vi "Handle Error.vi"(8 "error in (no error)":errorcluster, 11 "BNT_DAQmx-MCSV-AIAvg in":refnum<class "BNT_DAQmx-MCSV-AIAvg.lvclass">) -> (0 "error out":errorcluster, 2 "stop actor?":bool=TRUE, 3 "BNT_DAQmx-MCSV-AIAvg out":refnum<class "BNT_DAQmx-MCSV-AIAvg.lvclass">)   [LabVIEW 2019, in "BNT_DAQmx.lvlib" / "BNT_DAQmx-MCSV-AIAvg.lvclass"]
doc: "(<B>Filename</B>: Actor Framework.lvlib:Actor.lvclass:Handle Error.vi)\n\nDefines how the actor handles an error that occurred while processing a message.\n\nBy default, this method does nothing except stop the actor. This method also treats error code 43 (coming from <B>error in</B>) as a sign that the actor shut down normally. In this situation, the Handle Error method does not return the error on <B>error out</B>, meaning the actor's caller will not receive it. All other error codes will be returned on <B>error out</B>.\n\nA descendant class may override this method to change this behavior."
uses:
  BNT_DAQmx-MCSV-AIAvg.lvclass
  C:/User/Brand/LVP/TASCA/UTCS/Packages/CSPP_Core/Actors/CSPP_BaseActor/CSPP_BaseActor.lvclass
  CSPP_Core/Actors/CSPP_BaseActor/CSPP_BaseActor.lvclass/CSPP_BaseActor.ctl
  CSPP_Core/Libraries/Base/Severity.ctl
  BNT_DAQmx-MCSV/BNT_DAQmx-MCSV.lvclass
  CSPP_Core/Libraries/Base/CSPP_Base.lvlib
  CSPP_Core/Libraries/Utilities/CSPP_Utilities.lvlib
  CSPP_Core/Actors/CSPP_BaseActor/CSPP_BaseActor.lvclass
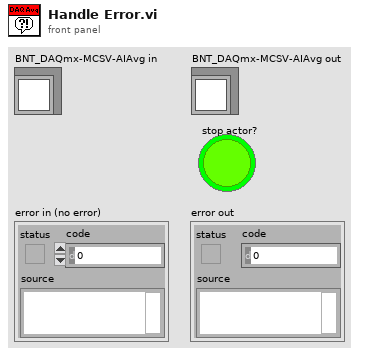
[diagram p1: front panel]
types:
  T1 = typedef "CSPP_Base.lvlib/Severity.ctl" = enum16{"emergency", "alert", "critical", "error", "warning", "notice", "info", "debug"}
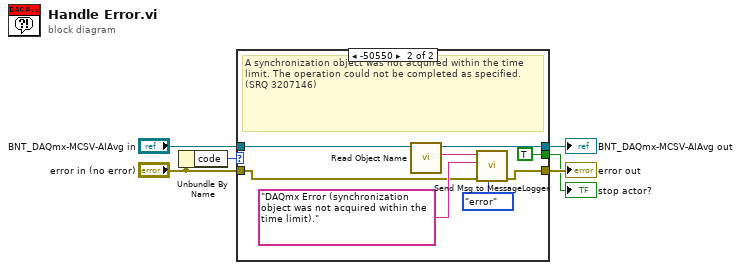
[diagram p0: block diagram]
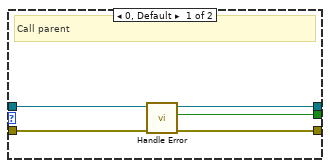
[diagram p2: hidden frame]
diagram:
  n1 = Unbundle By Name("error in (no error)") -> ("code"=w1:i32)
  n2 = case shown="-50550" w1 {
    tunnel: [w11 w13] -> w6
    tunnel: [w10 TRUE ("stop actor?")] -> w5
    tunnel: [w9 w15] -> w4
    tunnel: "error in (no error)" -> [w8 w14]
    tunnel: "BNT_DAQmx-MCSV-AIAvg in" -> [w7 w16]
    frame 0, Default {
      # "Call parent"
      n3 = call-parent "Handle Error.vi"("error in (no error)"=w8, "CSPP_BaseActor in"=w7) -> ("error out"=w11:errorcluster, "stop actor?"=w10:bool, "CSPP_BaseActor out"=w9:refnum<class "BNT_DAQmx-MCSV-AIAvg.lvclass">)  [unwired: 7 in]
    }
    frame -50550 {
      # "A synchronization object was not acquired within the time limit. The operation could not be completed as specified. (SRQ 3207146)"
      n4 = call "Read Object Name.vi"("CSPP_BaseActor in"=w16) -> ("Object Name"=w19:string, "CSPP_BaseActor out"=w15:refnum<class "BNT_DAQmx-MCSV-AIAvg.lvclass">)  [unwired: 8 in, 1 out]
      n5 = call "Send Msg to MessageLogger.vi"("Severity Code (info)"=Severity."error", "Error In"=w14, "Message Content"="DAQmx Error (synchronization object was not acquired within the time limit).", "Message Tag"=w19) -> ("Error Out"=w13:errorcluster)  [unwired: 7 in]
    }
  }
  "BNT_DAQmx-MCSV-AIAvg out" <- w4
  "error out" <- w6
  "stop actor?" <- w5
